vi "Config BERT Data.vi"(0 "VISA Resource Name":refnum<visa-resource-name>, 1 "Data (T:PN9)":bool=TRUE, 2 "Max Data Rate (T:2Mbps)":bool=TRUE, 3 "Total Bits (10000)":i32=10000, 5 "error in (no error)":errorcluster {"code" format="%.0x"}, 6 "Special Pattern Ignore (F:OFF)":bool, 8 "Special Pattern (T:0's)":bool=TRUE, 10 "BERT Resync (F:OFF)":bool, 12 "Resync Limits (0.4000)":dbl=0.4 format="%.4f") -> (14 "VISA Resource Name Out":refnum<visa-resource-name>, 19 "error out":errorcluster {"code" format="%.0x"})   [LabVIEW 2014, in "Agilent ESG Series.lvlib"]
doc: "This VI is used to configure the CDMA option.\n\nThis VI is valid only on instruments with the UND and UN5 options."
uses:
  Agilent ESG Series.lvlib
panel:
  # "2Mbps"
  # "PN9"
  # "10Mbps"
  # "PN15"
  # "ON"
  # "OFF"
  # "0's"
  # "ON"
  # "OFF"
  # "1's"
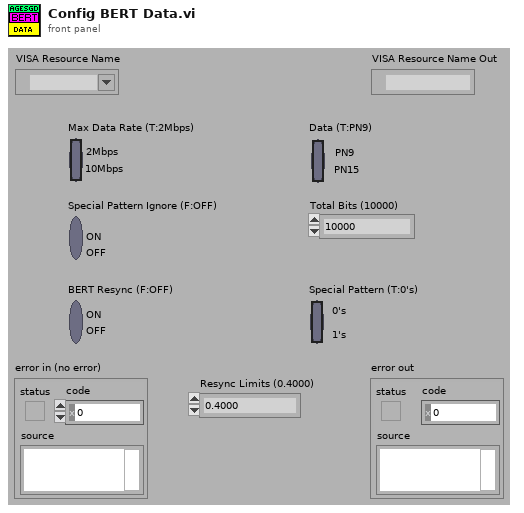
[diagram p1: front panel]
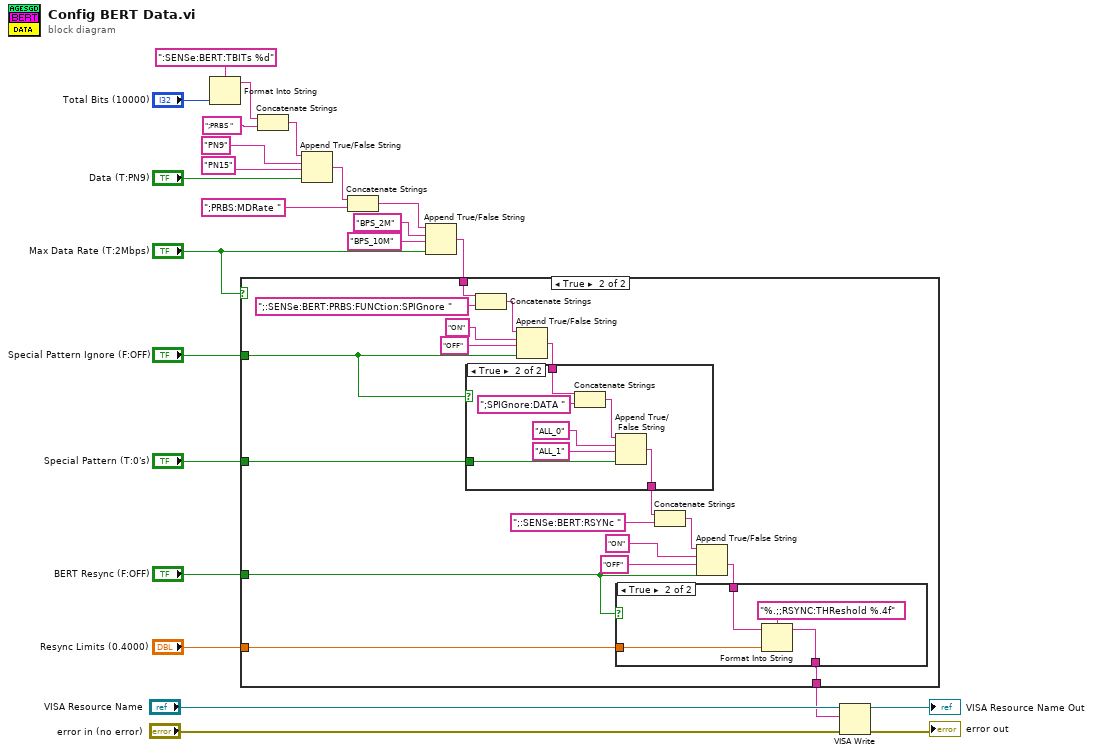
[diagram p0: block diagram]
diagram:
  n1 = Format Into String(format string=":SENSe:BERT:TBITs %d", "Total Bits (10000)") -> (resulting string=w10:string)  [unwired: 2 in, 1 out]
  n2 = Concatenate Strings(w10, ";PRBS " ("string (\"\")")) -> (w8:string)
  n3 = Append True/False String(1:"Data (T:PN9)", 2:"PN15" ("false string"), 3:"PN9" ("true string"), 4:w8) -> (0:w11:string)
  n4 = Concatenate Strings(w11, ";PRBS:MDRate ") -> (w13:string)
  n5 = Append True/False String(1:"Max Data Rate (T:2Mbps)", 2:"BPS_10M" ("false string"), 3:"BPS_2M" ("true string"), 4:w13) -> (0:w7:string)
  n6 = case shown="True" "Max Data Rate (T:2Mbps)" {
    tunnel: w7 -> [w25 w39]
    tunnel: "Special Pattern Ignore (F:OFF)" -> [_ w38]
    tunnel: "BERT Resync (F:OFF)" -> [_ w32]
    tunnel: "Resync Limits (0.4000)" -> [_ w31]
    tunnel: [w25 w29] -> w1
    tunnel: "Special Pattern (T:0's)" -> [_ w28]
    frame False {
    }
    frame True {
      n7 = Concatenate Strings(w39, ";:SENSe:BERT:PRBS:FUNCtion:SPIGnore ") -> (w26:string)
      n8 = Append True/False String(1:w38, 2:"OFF" ("false string"), 3:"ON" ("true string"), 4:w26) -> (0:w27:string)
      n9 = case shown="True" w38 {
        tunnel: [w48 w51] -> w30
        tunnel: w28 -> [_ w50]
        tunnel: w27 -> [w48 w49]
        frame False {
        }
        frame True {
          n10 = Concatenate Strings(w49, ";SPIGnore:DATA ") -> (w53:string)
          n11 = Append True/False String(1:w50, 2:"ALL_1" ("false string"), 3:"ALL_0" ("true string"), 4:w53) -> (0:w51:string)
        }
      }
      n12 = Concatenate Strings(w30, ";:SENSe:BERT:RSYNc ") -> (w35:string)
      n13 = Append True/False String(1:w32, 2:"OFF" ("false string"), 3:"ON" ("true string"), 4:w35) -> (0:w33:string)
      n14 = case shown="True" w32 {
        tunnel: w33 -> [w43 w46]
        tunnel: w31 -> [_ w47]
        tunnel: [w43 w44] -> w29
        frame False {
        }
        frame True {
          n15 = Format Into String(format string="%.;;RSYNC:THReshold %.4f" ("true string"), initial string=w46, w47) -> (resulting string=w44:string)  [unwired: 1 in, 1 out]
        }
      }
    }
  }
  n16 = VISA Write(VISA resource name="VISA Resource Name", write buffer=w1, error in (no error)="error in (no error)") -> (VISA resource name out=→"VISA Resource Name Out":refnum<visa-resource-name>, error out=→"error out":errorcluster)  [unwired: 1 out]
